vi "Lichtansteuerung.vi"(8 "error in (no error)":errorcluster caption="Fehler (Eingang, kein Fehler)", 11 "Device ID":T1(ring)) -> (0 "error out":errorcluster caption="Fehler (Ausgang)", 3 "Device ID Out":T1(ring))   [LabVIEW 2010]
uses:
  sub VIs v Hauptprogramm/globale Variable 1.vi
panel:
  out "error out 2":errorcluster
  out "True?":bool
  in  "Seite2":dbl
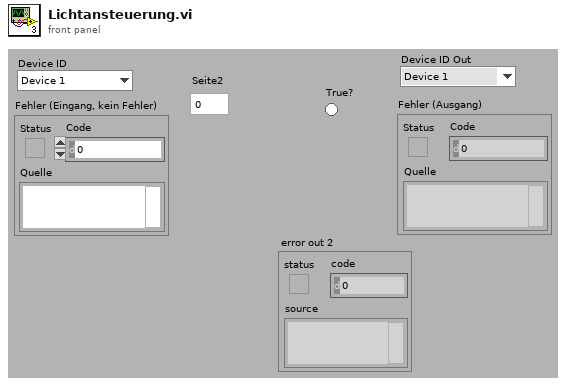
[diagram p1: front panel]
types:
  T1 = enum16{"Device 1", "Device 2", "Device 3", "Device 4", "Device 5", "Device 6", "Device 7", "Device 8"}
  T2 = enum8{"Input 1 (I1)", "Input 2 (I2)", "Input 3 (I3)", "Input 4 (I4)", "Input 5 (I5)", "Input 6 (I6)", "Input 7 (I7)", "Input 8 (I8)"}
  T3 = enum8{"Robo Interface", "Extension 1", "Extension 2", "Extension 3"}
  T4 = enum8{"Power 1", "Power 2", "Power 3", "Power 4", "Power 5", "Power 6", "Power 7", "Power 8"}
  T5 = enum8{"Output 1 (O1)", "Output 2 (O2)", "Output 3 (O3)", "Output 4 (O4)", "Output 5 (O5)", "Output 6 (O6)", "Output 7 (O7)", "Output 8 (O8)"}
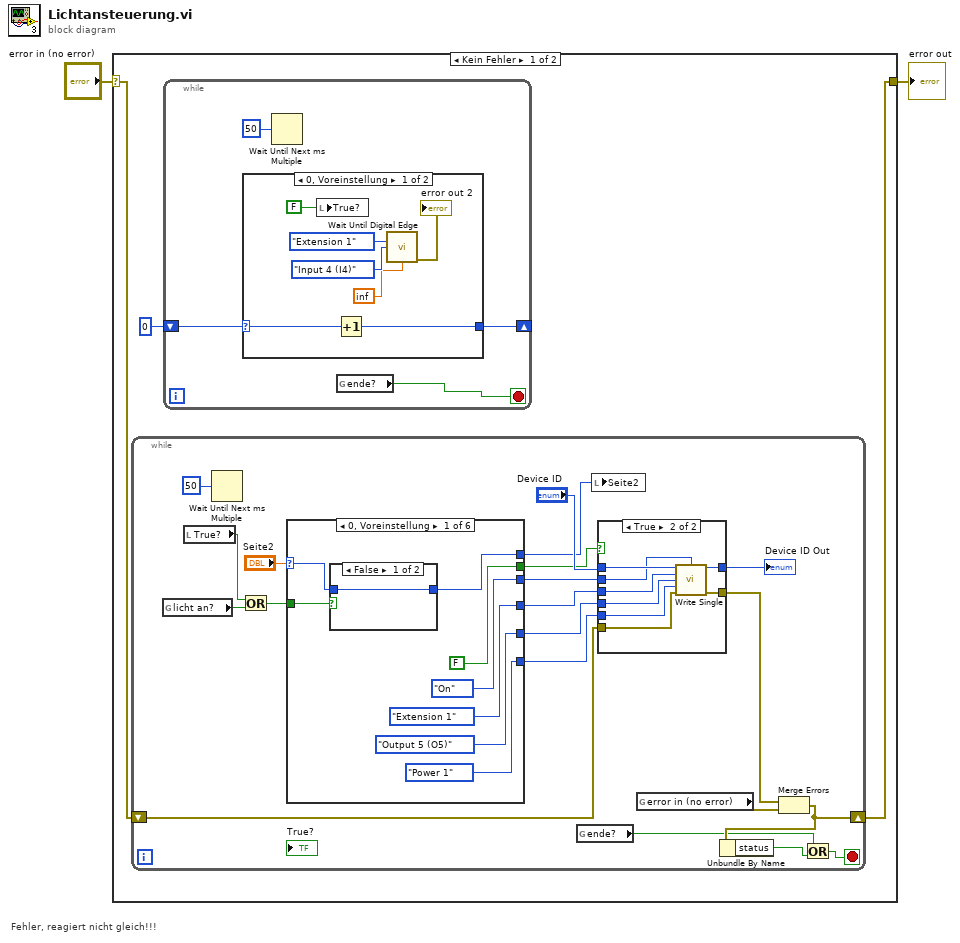
[diagram p0: block diagram]
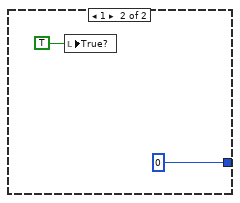
[diagram p2: hidden frame]
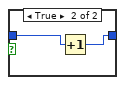
[diagram p3: hidden frame]
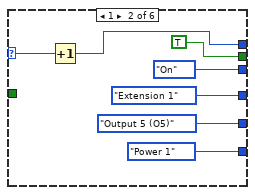
[diagram p4: hidden frame]
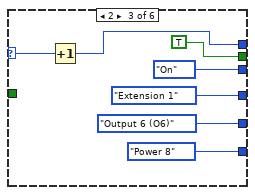
[diagram p5: hidden frame]
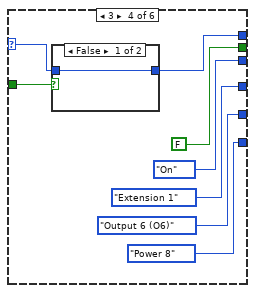
[diagram p6: hidden frame]
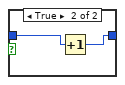
[diagram p7: hidden frame]
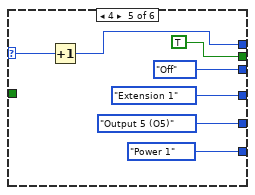
[diagram p8: hidden frame]
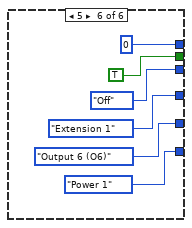
[diagram p9: hidden frame]
diagram:
  # "Fehler, reagiert nicht gleich!!!"
  n1 = case shown="Kein Fehler" "error in (no error)" {
    selector: "error in (no error)" -> [w4 w98]
    tunnel: [w5 w98] -> w2
    frame No Error {
      n2 = while {
        shift-right: [w22] -> w5
        shift-left: w4 -> [w26]
        stop <- w21 stop-if-true
        n3 = global read "globale Variable 1.vi" "licht an?"() -> (w33:bool)
        n4 = local read "True?"() -> (w34:bool)
        n5 = Wait Until Next ms Multiple(millisecond multiple=50) -> ()  [unwired: 1 out]
        n6 = Or(x=w34, y=w33) -> (x .or. y?=w32:bool)
        n7 = case shown="0, Voreinstellung" "Seite2" {
          selector: "Seite2" -> [w45 w56 w63 w66 w76 _]
          tunnel: [w44 w55 w62 w65 w75 0] -> w35
          tunnel: w32 -> [w46 _ _ w64 _ _]
          tunnel: [FALSE TRUE TRUE FALSE TRUE TRUE] -> w31
          tunnel: [enum8{"Off", "On"}."On" ("Output_Action") enum8{"Off", "On"}."On" ("Output_Action") enum8{"Off", "On"}."On" ("Output_Action") enum8{"Off", "On"}."On" ("Output_Action") enum8{"Off", "On"}."Off" ("Output_Action") enum8{"Off", "On"}."Off" ("Output_Action")] -> w30
          tunnel: [T3."Extension 1" ("Module") T3."Extension 1" ("Module") T3."Extension 1" ("Module") T3."Extension 1" ("Module") T3."Extension 1" ("Module") T3."Extension 1" ("Module")] -> w29
          tunnel: [T5."Output 5 (O5)" ("Single_Output") T5."Output 5 (O5)" ("Single_Output") T5."Output 6 (O6)" ("Single_Output") T5."Output 6 (O6)" ("Single_Output") T5."Output 5 (O5)" ("Single_Output") T5."Output 6 (O6)" ("Single_Output")] -> w28
          tunnel: [T4."Power 1" ("Output_PWM") T4."Power 1" ("Output_PWM") T4."Power 8" ("Output_PWM") T4."Power 8" ("Output_PWM") T4."Power 1" ("Output_PWM") T4."Power 1" ("Output_PWM")] -> w27
          frame 0, Default {
            n8 = case shown="FALSE" w46 {
              tunnel: w45 -> [w47 w49]
              tunnel: [w47 w48] -> w44
              frame False {
              }
              frame True {
                n9 = Increment(x=w49) -> (x+1=w48:i32)
              }
            }
          }
          frame 1 {
            n10 = Increment(x=w56) -> (x+1=w55:i32)
          }
          frame 2 {
            n11 = Increment(x=w63) -> (x+1=w62:i32)
          }
          frame 3 {
            n12 = case shown="FALSE" w64 {
              tunnel: w66 -> [w72 w74]
              tunnel: [w72 w73] -> w65
              frame False {
              }
              frame True {
                n13 = Increment(x=w74) -> (x+1=w73:i32)
              }
            }
          }
          frame 4 {
            n14 = Increment(x=w76) -> (x+1=w75:i32)
          }
          frame 5 {
          }
        }
        n15 = global read "globale Variable 1.vi" "ende?"() -> (w19:bool)
        n16 = local write "Seite2"(w35) -> ()
        n17 = case shown="TRUE" w31 {
          tunnel: [w89 w96] -> w38
          tunnel: [w88 w97] -> w25
          tunnel: "Device ID" -> [w89 w95]
          tunnel: w30 -> [_ w94]
          tunnel: w29 -> [_ w93]
          tunnel: w28 -> [_ w92]
          tunnel: w27 -> [_ w91]
          tunnel: w26 -> [w88 w90]
          frame False {
          }
          frame True {
            n18 = call "Write Single.vi"("Device ID"=w95, "Output_Action"=w94, "Module"=w93, "Single_Output"=w92, "Output_PWM"=w91, "error in"=w90) -> ("Device ID Out"=w96:T1, "error out"=w97:errorcluster)  [unwired: 8 out]
          }
        }
        "Device ID Out" <- w38
        n19 = global read "globale Variable 1.vi" "error in (no error)"() -> (w24:errorcluster)
        n20 = Merge Errors(w25, w24) -> (w22:errorcluster)
        n21 = Unbundle By Name(w22) -> ("status"=w20:bool)
        n22 = Or(x=w19, y=w20) -> (x .or. y?=w21:bool)
      }
      n23 = while {
        shift-right: [w7] -> _
        shift-left: 0 -> [w8]
        stop <- w6 stop-if-true
        n24 = case shown="0, Voreinstellung" w8 {
          selector: w8 -> [w14 _]
          tunnel: [w13 0] -> w7
          frame 0, Default {
            n25 = local write "True?"(FALSE ("True?")) -> ()
            n26 = Increment(x=w14) -> (x+1=w13:i32)
            n27 = call "Wait Until Digital Edge.vi"("Module"=T3."Extension 1", "Digital_Input"=T2."Input 4 (I4)", "Time Out (10)"=inf) -> ("error out"=→"error out 2":errorcluster)  [unwired: 3 in, 9 out]
          }
          frame 1 {
            n28 = local write "True?"(TRUE ("True?")) -> ()
          }
        }
        n29 = Wait Until Next ms Multiple(millisecond multiple=50) -> ()  [unwired: 1 out]
        n30 = global read "globale Variable 1.vi" "ende?"() -> (w6:bool)
      }
    }
    frame Error {
    }
  }
  "error out" <- w2
